vi "Clear-diplays.vi"(8 "error in":errorcluster, 11 "UI ref. in":refnum<data-value>) -> (0 "error IO":errorcluster, 3 "UI ref.":refnum<data-value>)   [LabVIEW 2013, in "CameraVision.lvlib" / "CV-UI.lvclass"]
doc: "This function deletes the data from the various GUI graphs and displays. This avoids interference with data from a previous acquisition."
uses:
  CV-UI.lvclass
  Display-names.ctl
  CV-UI.lvclass/CV-UI.ctl
  Read Display refs.vi
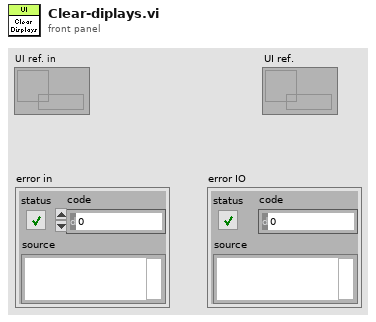
[diagram p1: front panel]
types:
  T1 = typedef "CameraVision.lvlib/CV-UI.lvclass/Display-names.ctl" = enum16{"State", "Action", "Current image", "Framerate", "Frametime", "Process buffer", "Storage buffer", "Free disk space", "Total disk space", "Information", "Histogram", "Camera 1", "Camera 2", "Camera 1 chart", "Camera 2 chart", "Browser", "Temperature", "Map", "Status overview", "Characteristics", "Temper characteristics"}
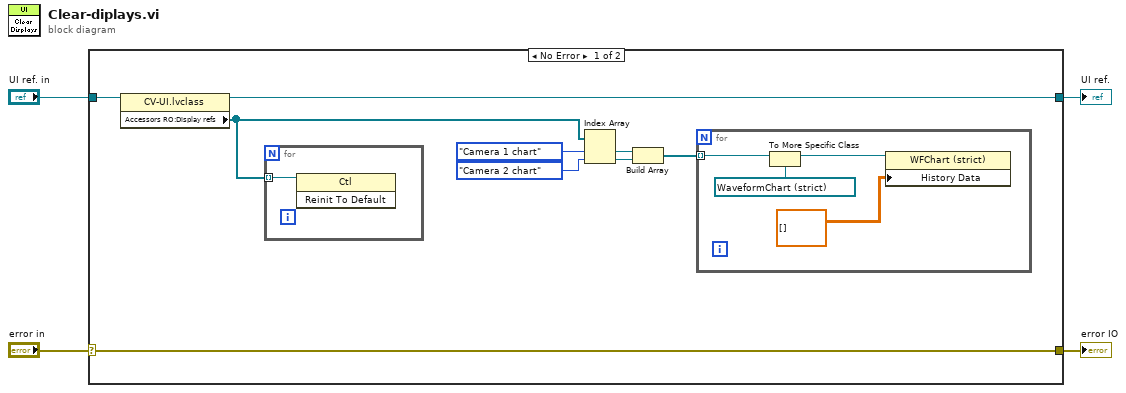
[diagram p0: block diagram]
diagram:
  n1 = case shown="No Error" "error in" {
    selector: "error in" -> [w13 w20]
    tunnel: [w13 w20] -> w4
    tunnel: "UI ref. in" -> [w6 w19]
    tunnel: [w5 w19] -> w1
    frame No Error {
      n2 = property class="CV-UI.lvclass"(reference=w6) -> (reference out=w5:refnum<data-value>, "Accessors RO:Display refs"=w12:refnum<vi>[])  [unwired: 1 in, 1 out]
      n3 = for {
        tunnel: w12 -> [w18] mode=indexing
        n4 = invoke class="Ctl" method="Reinit To Default"(reference=w18) -> ()  [unwired: 2 in, 3 out]
      }
      n5 = Index Array(array=w12, index #1=Display-names."Camera 1 chart" ("Dislay"), index #2=Display-names."Camera 2 chart" ("Dislay")) -> (element #1=w9:refnum<vi>, element #2=w8:refnum<vi>)
      n6 = Build Array(w9, w8) -> (w7:refnum<vi>[])
      n7 = for {
        tunnel: w7 -> [w17] mode=indexing
        n8 = To More Specific Class(target class=refnum<vi> refnum ("Cam. 1 chart"), reference=w17) -> (specific class reference=w15:refnum<vi>)  [unwired: 1 in, 1 out]
        n9 = property on="Property Node" class="WFChart (strict)"(reference=w15, "History Data"=dbl[][] []) -> ()  [unwired: 1 in, 2 out]
      }
    }
    frame Error {
    }
  }
  "error IO" <- w4
  "UI ref." <- w1
